vi "Introspection Core.vi"(8 "error in (no error)":errorcluster, 11 "CS++DSCManager in":refnum<class "CS++DSCManager.lvclass">) -> (0 "error out":errorcluster, 2 "CS++Messages":refnum<class "Message.lvclass">[](array[class]), 3 "CS++DSCManager out":refnum<class "CS++DSCManager.lvclass">)   [LabVIEW 2014, in "CS++DSCManager.lvlib" / "CS++DSCManager.lvclass"]
doc: "This vi delivers a list with all messages this actor reacts to. \n\nNote that all inherited classes have to overwrite it."
uses:
  CS++DSCManager.lvclass
  <vilib>/ActorFramework/Message/Message.lvclass
  CS++DSCManager Messages/Deploy Libraries Msg/Deploy Libraries Msg.lvclass
  CS++DSCManager Messages/Save Process to Library Msg/Save Process to Library Msg.lvclass
  CS++DSCManager Messages/Save SV to Library Msg/Save SV to Library Msg.lvclass
  CS++DSCManager Messages/Undeploy Libraries Msg/Undeploy Libraries Msg.lvclass
  CS++DSCManager Messages/Create Process Msg/Create Process Msg.lvclass
  CS++DSCManager Messages/Enable Process Msg/Enable Process Msg.lvclass
  CS++DSCManager Messages/Enable Process Alarm Logging Msg/Enable Process Alarm Logging Msg.lvclass
  CS++DSCManager Messages/Enable Process Data Logging Msg/Enable Process Data Logging Msg.lvclass
  CS++DSCManager Messages/Delete Process Msg/Delete Process Msg.lvclass
  CS++DSCManager Messages/Create SV Msg/Create SV Msg.lvclass
  CSPP_Core/Actors/CS++BaseActor/CS++BaseActor.lvclass
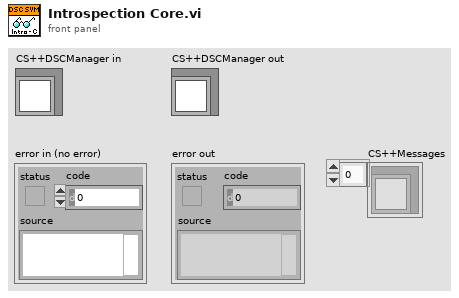
[diagram p1: front panel]
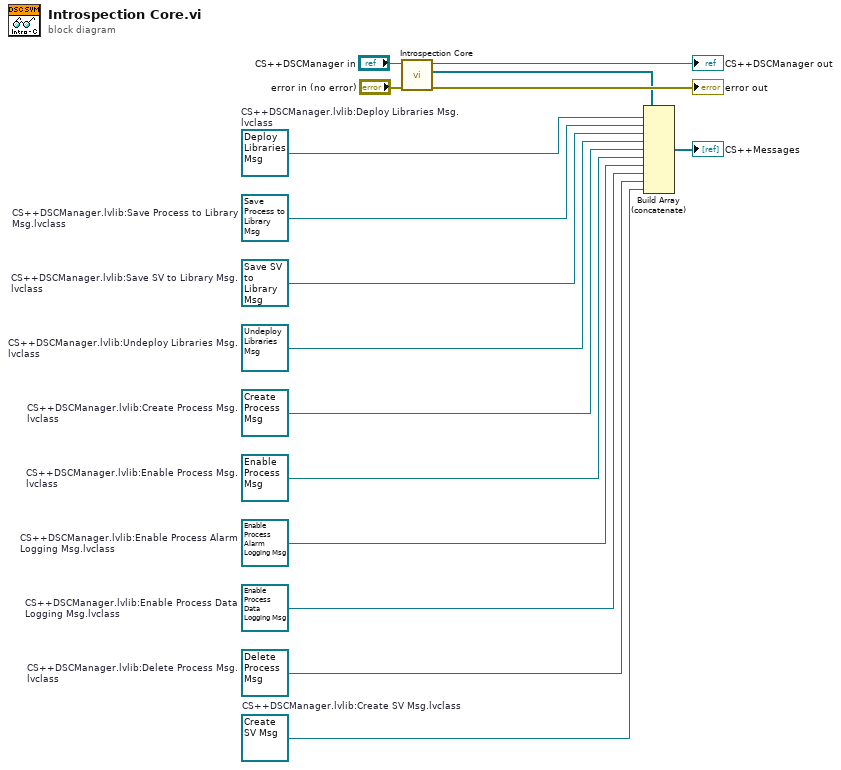
[diagram p0: block diagram]
diagram:
  w1 = refnum<class "Create SV Msg.lvclass"> refnum  # CS++DSCManager.lvlib:Create SV Msg.lvclass
  w2 = refnum<class "Delete Process Msg.lvclass"> refnum  # CS++DSCManager.lvlib:Delete Process Msg.lvclass
  w3 = refnum<class "Enable Process Data Logging Msg.lvclass"> refnum  # CS++DSCManager.lvlib:Enable Process Data Logging Msg.lvclass
  w4 = refnum<class "Enable Process Alarm Logging Msg.lvclass"> refnum  # CS++DSCManager.lvlib:Enable Process Alarm Logging Msg.lvclass
  w5 = refnum<class "Enable Process Msg.lvclass"> refnum  # CS++DSCManager.lvlib:Enable Process Msg.lvclass
  w6 = refnum<class "Create Process Msg.lvclass"> refnum  # CS++DSCManager.lvlib:Create Process Msg.lvclass
  w7 = refnum<class "Undeploy Libraries Msg.lvclass"> refnum  # CS++DSCManager.lvlib:Undeploy Libraries Msg.lvclass
  w8 = refnum<class "Save SV to Library Msg.lvclass"> refnum  # CS++DSCManager.lvlib:Save SV to Library Msg.lvclass
  w9 = refnum<class "Save Process to Library Msg.lvclass"> refnum  # CS++DSCManager.lvlib:Save Process to Library Msg.lvclass
  w10 = refnum<class "Deploy Libraries Msg.lvclass"> refnum  # CS++DSCManager.lvlib:Deploy Libraries Msg.lvclass
  n1 = call-parent "Introspection Core.vi"("error in (no error)"="error in (no error)", "CS++BaseActor in"="CS++DSCManager in") -> ("error out"=→"error out":errorcluster, "CS++Messages"=w15:refnum<class "Message.lvclass">[], "CS++BaseActor out"=→"CS++DSCManager out":refnum<class "CS++DSCManager.lvclass">)  [unwired: 7 in]
  n2 = Build Array (concatenate)(w15, w10, w9, w8, w7, w6, w5, w4, w3, w2, w1) -> (→"CS++Messages":refnum<class "Message.lvclass">[])
